vi "StringTag.value_lua.vi"(5 "LuaVIEW reference":T1) -> (15 "error out":errorcluster)   [LabVIEW 2012]
doc: "Returns the current value of a string tag. This equals the last string written to the tag. On initialisation, the datalogger rebuffers the last string which is therefore guaranteed to be available without requiring disk I/O.\nParameters:\nobj:strtag\nResults:\nstr:value, last written string.\nErrors:\nDead or invalid tag object.\nData logger not initialized."
uses:
  luaview/typedefs/t_LuaVIEW Reference.ctl
  typedefs/t_DataLog Live Tag Strings Methods.ctl
  luaview/subvis/private/LuaVIEW Pull (object).vi
  luaview/subvis/private/LuaVIEW Push (string).vi
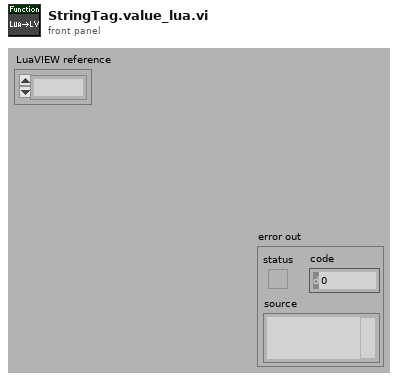
[diagram p1: front panel]
types:
  T1 = typedef "t_LuaVIEW Reference.ctl" = refnum<k1>
  T2 = typedef "t_DataLog Live Tag Strings Methods.ctl" = enum16{"initialize", "rebuffer", "read", "write", "cleanup"}
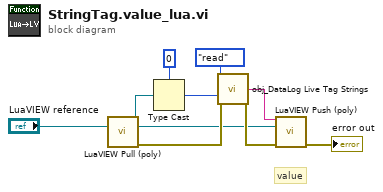
[diagram p0: block diagram]
diagram:
  # "value"
  n1 = call-poly "LuaVIEW Pull (poly).vi"("LuaVIEW reference in"="LuaVIEW reference") -> ("object refnum"=w10:refnum<vi>, "LuaVIEW reference out"=w2:T1, "error out"=w6:errorcluster)  [unwired: 11 in, 1 out]
  n2 = Type Cast(type=0 ("read index in"), x=w10) -> (*(type *) &x=w5:i32)
  n3 = call "obj_DataLog Live Tag Strings.vi"("method"=t_DataLog_Live_Tag_Strings_Methods."read", "tag index"=w5, "error in (no error)"=w6) -> ("string out"=w3:string, "error out"=w4:errorcluster)  [unwired: 9 in, 2 out]
  n4 = call-poly "LuaVIEW Push (poly).vi"("string"=w3, "LuaVIEW reference in"=w2, "error in (no error)"=w4) -> ("error out"=→"error out":errorcluster)  [unwired: 11 in, 1 out]
